vi "Construct Client Controller.vi"(8 "error in (no error)":errorcluster, 10 "Base Path":path) -> (0 "error out":errorcluster, 3 "Client Controller out":refnum<class "Client Controller.lvclass">)   [LabVIEW 2015, in "Client Controller.lvlib" / "Client Controller.lvclass"]
uses:
  Client Controller.lvclass
  UI/Client UI.lvclass
  Client Config.lvclass
  <userlib>/Common Components/Controller/Controller.lvclass/Controller.ctl
  <userlib>/Common Components/Controller/Accessors/Write Root Path.vi
  <userlib>/Common Components/Controller/Controller.lvclass
  <userlib>/Configuration Dialog Actor/Configuration.lvclass
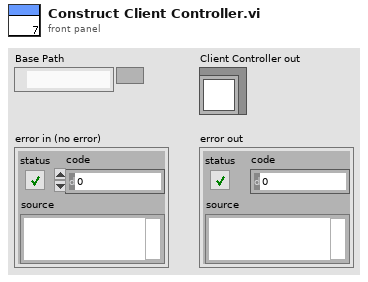
[diagram p1: front panel]
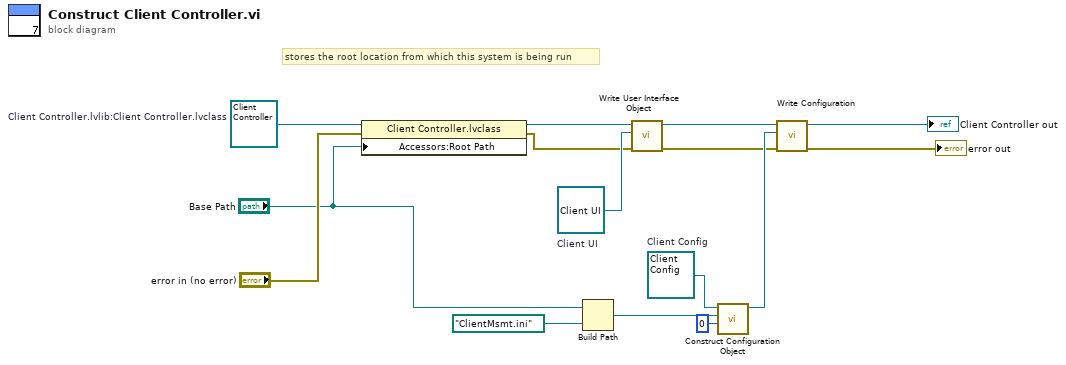
[diagram p0: block diagram]
diagram:
  w14 = refnum<class "Client Config.lvclass"> refnum  # Client Config
  w9 = refnum<class "Client UI.lvclass"> refnum  # Client UI
  w8 = refnum<class "Client Controller.lvclass"> refnum  # Client Controller.lvlib:Client Controller.lvclass
  # "stores the root location from which this system is being run"
  n1 = property class="Client Controller.lvclass"(reference=w8, error in="error in (no error)", "Accessors:Root Path"="Base Path") -> (reference out=w7:refnum<class "Client Controller.lvclass">, error out=w5:errorcluster)
  n2 = Build Path(base path="Base Path", name or relative path=path "ClientMsmt.ini" ("Base Path")) -> (appended path=w3:path)
  n3 = call <userlib>:"Write User Interface Object.vi"("error in (no error)"=w5, "UI.lvclass"=w9, "UI Controller in"=w7) -> ("error out"=w11:errorcluster, "UI Controller out"=w10:refnum<class "Client Controller.lvclass">)  [unwired: 7 in]
  n4 = call <userlib>:"Construct Configuration Object.vi"("Initial Category Selection"=0, "Configuration File Path"=w3, "Configuration in"=w14) -> ("Configuration out"=w15:refnum<class "Client Config.lvclass">)  [unwired: 5 in, 3 out]
  n5 = call <userlib>:"Write Configuration.vi"("error in (no error)"=w11, "Configuration.lvlib:Configuration.lvclass"=w15, "Controller in"=w10) -> ("error out"=→"error out":errorcluster, "Controller out"=→"Client Controller out":refnum<class "Client Controller.lvclass">)  [unwired: 7 in]
